vi "INTELLIFAUCET Linear Interpolation GPMtouA.vi"(8 "Error In":errorcluster, 10 "Target":dbl, 11 "Interpolation Table(Xs,Ys)":dbl[][](array[numeric])=[[23.0, 6000.0], [37.0, 8400.0]]) -> (0 "Error Out":errorcluster, 2 "uA Output":i32)   [LabVIEW 2016]
uses:
  <vilib>/gmath/NI_Gmath.lvlib
panel:
  # "Need to add calibration file to fine tune this. Will make responcse better on the PID....or build conversion sheet during first purge"
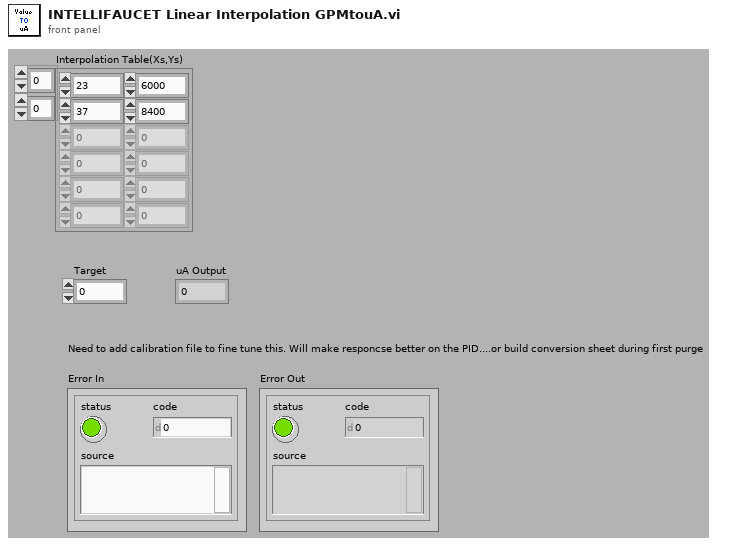
[diagram p1: front panel]
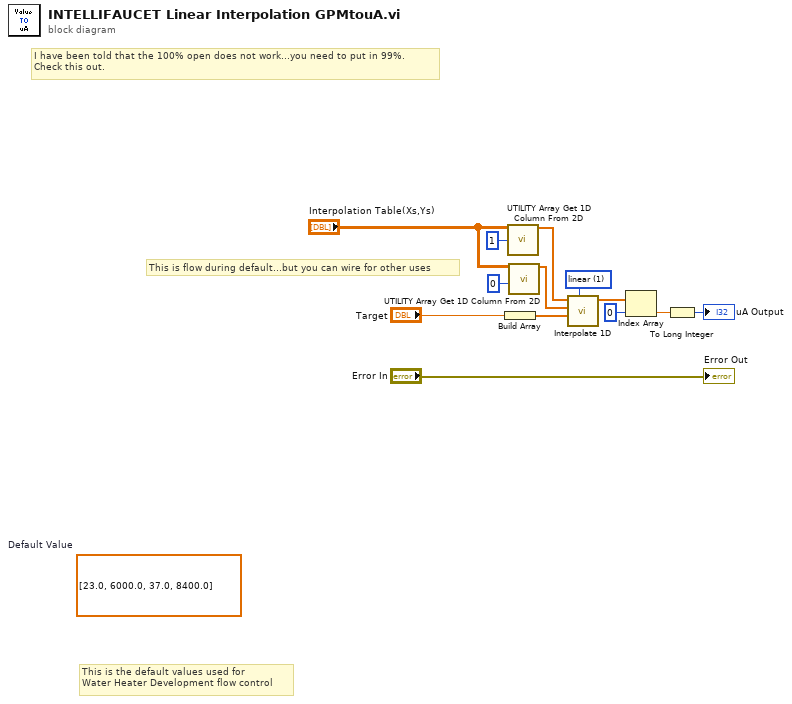
[diagram p0: block diagram]
diagram:
  (unwired) dbl[][] [[23.0, 6000.0], [37.0, 8400.0]]  # Default Value
  w12 = 1 items=["nearest", "linear", "spline", "cubic Hermite", "Lagrange"] ("method")
  # "This is the default values used for \nWater Heater Development flow control"
  # "I have been told that the 100% open does not work...you need to put in 99%. \nCheck this out."
  # "This is flow during default...but you can wire for other uses"
  n1 = Build Array("Target") -> (w9:dbl[])
  n2 = call "UTILITY Array Get 1D Column From 2D.vi"("2D Array Data"="Interpolation Table(Xs,Ys)", "column index"=1) -> ("Column Data"=w3:dbl[])  [unwired: 13 in]
  n3 = call "UTILITY Array Get 1D Column From 2D.vi"("2D Array Data"="Interpolation Table(Xs,Ys)", "column index"=0) -> ("Column Data"=w4:dbl[])  [unwired: 13 in]
  n4 = call <vilib>:"Interpolate 1D.vi"("method"=w12, "xi"=w9, "X"=w4, "Y"=w3) -> ("yi"=w8:dbl[])  [unwired: 5 in, 2 out]
  n5 = Index Array(array=w8, index=0) -> (element=w5:dbl)
  n6 = To Long Integer(number=w5) -> (32bit integer=→"uA Output":i32)
  "Error Out" <- "Error In"
